vi "D6_Root path.vi"(8 "error in (no error)":errorcluster) -> (0 "error out":errorcluster, 3 "Root Path":T1)   [LabVIEW 2022 SP3]
uses:
  Controls/D6 Root path.ctl
panel:
  out "appended path":path
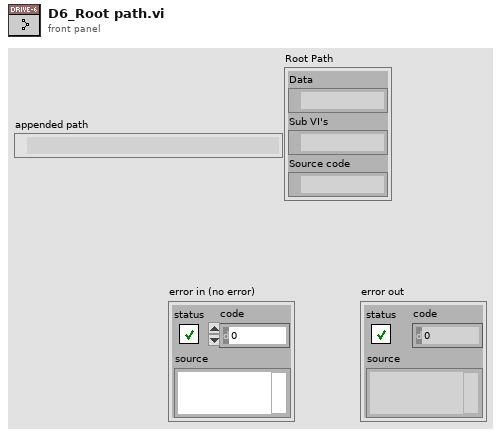
[diagram p1: front panel]
types:
  T1 = typedef "D6 Root path.ctl" = cluster{"Data":path, "Sub VI's":path, "Source code":path}
  T2 = enum32{"invalid app kind", "Development System", "Run Time System", "Student Edition", "Embedded LabVIEW", "Evaluation", "Custom"}
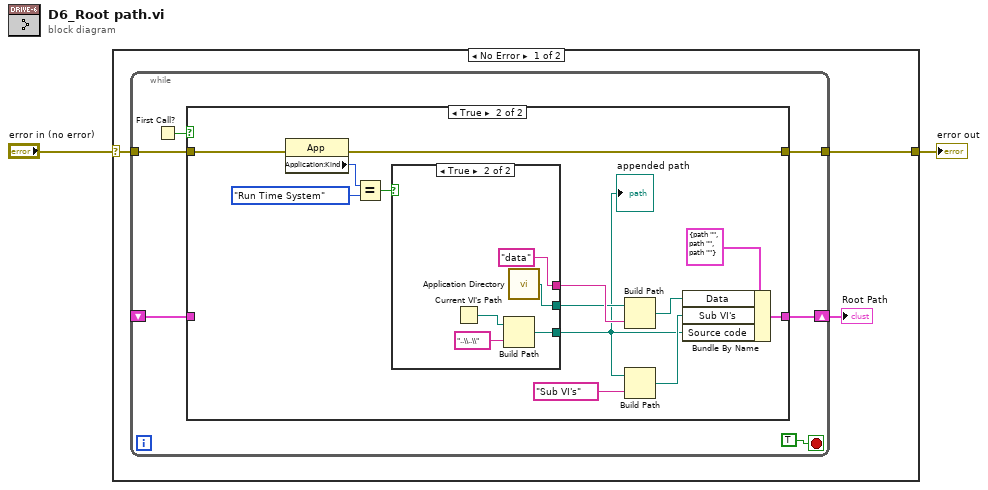
[diagram p0: block diagram]
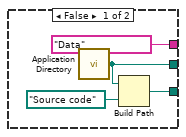
[diagram p3: hidden frame]
diagram:
  n1 = case shown="No Error" "error in (no error)" {
    selector: "error in (no error)" -> [w5 w36]
    tunnel: [w4 w36] -> w1
    frame No Error {
      n2 = while {
        tunnel: w5 -> [w8]
        tunnel: [w10] -> w4
        shift-right: [w7] -> w3
        shift-left: _ -> [w6]
        stop <- TRUE stop-if-true
        n3 = First Call?() -> (First Call?: T/F=w11:bool)
        n4 = case shown="True" w11 {
          tunnel: w8 -> [w13 w23]
          tunnel: [w13 w22] -> w10
          tunnel: [w12 w17] -> w7
          tunnel: w6 -> [w12 _]
          frame False {
            # "Get Paths"
          }
          frame True {
            n5 = property class="App"(error in=w23) -> (error out=w22:errorcluster, "Application:Kind"=w26:T2)  [unwired: 1 in, 1 out]
            n6 = Equal?(x=w26, y=T2."Run Time System") -> (x = y?=w14:bool)
            n7 = case shown="True" w14 {
              tunnel: ["Data" ("name or relative path") "data" ("name or relative path")] -> w24
              tunnel: [w29 w33] -> w16
              tunnel: [w27 w31] -> w15
              frame False {
                n8 = call <vilib>:"Application Directory.vi"() -> ("Application Directory"=w29:path)
                n9 = Build Path(base path=w29, name or relative path=path "Source code") -> (appended path=w27:path)
              }
              frame True {
                n10 = Current VI's Path() -> (path=w35:path)
                n11 = Build Path(base path=w35, name or relative path="..\\..\\") -> (appended path=w31:path)
                n12 = call <vilib>:"Application Directory.vi"() -> ("Application Directory"=w33:path)
              }
            }
            "appended path" <- w15
            n13 = Build Path(base path=w16, name or relative path=w24) -> (appended path=w19:path)
            n14 = Build Path(base path=w15, name or relative path="Sub VI's") -> (appended path=w18:path)
            n15 = Bundle By Name(cluster=T1 {"Data"=path "", "Sub VI's"=path "", "Source code"=path ""} ("Root Path"), "Data"=w19, "Sub VI's"=w18, "Source code"=w15) -> (w17:T1)
          }
        }
      }
      "Root Path" <- w3
    }
    frame Error {
    }
  }
  "error out" <- w1
